vi "Clear_Trajectory.vi"(8 "error in (no error)":errorcluster) -> (0 "error out":errorcluster)   [LabVIEW 2019, in "Kinova MICO² USB.lvlib"]
uses:
  <vilib>/Utility/error.llb/Error Cluster From Error Code.vi
  <vilib>/ErrorRing/Error Ring.xnode
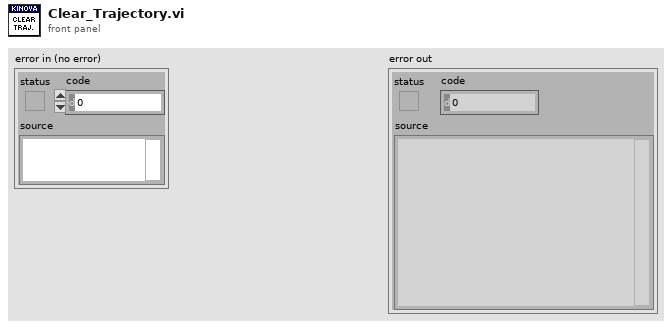
[diagram p1: front panel]
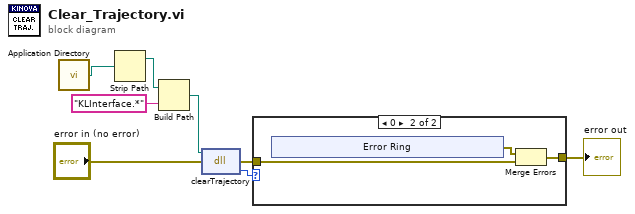
[diagram p0: block diagram]
diagram:
  n1 = call <vilib>:"Application Directory.vi"() -> ("Application Directory"=w1:path)
  n2 = Strip Path(path=w1) -> (stripped path=w5:path)  [unwired: 1 out]
  n3 = Build Path(base path=w5, name or relative path="KLInterface.*") -> (appended path=w2:path)
  n4 = dll-call lib="C:/Users/mcjssdcc/source/repos/Kinova Labview Interface/Debug/KLInterface.dll" fn="clearTrajectory"(path in=w2, error in="error in (no error)") -> (error out=w7:errorcluster, "return type"=w6:i32)  [unwired: 1 in, 1 out]
  n5 = case shown="0" w6 {
    tunnel: [w9 w11] -> w4
    tunnel: w7 -> [w9 w10]
    frame 1, Default {
    }
    frame 0 {
      n6 = xnode "Error Ring"() -> ("error out"=w12:errorcluster)
      n7 = Merge Errors(w12, w10) -> (w11:errorcluster)
    }
  }
  "error out" <- w4
